vi "Exp_PopulateADCQualityControl.vi"(8 "error in (no error)":errorcluster, 10 "Control":refnum<vi>, 11 "LightField Automation in":refnum<class "LightField Automation.lvclass">) -> (0 "error out":errorcluster, 3 "LightField Automation out":refnum<class "LightField Automation.lvclass">)   [LabVIEW 2020, in "LightField Automation.lvclass"]
uses:
  LightField Automation.lvclass
  C:/Program Files/Princeton Instruments/LightField/PrincetonInstruments.LightFieldAddInSupportServices.dll
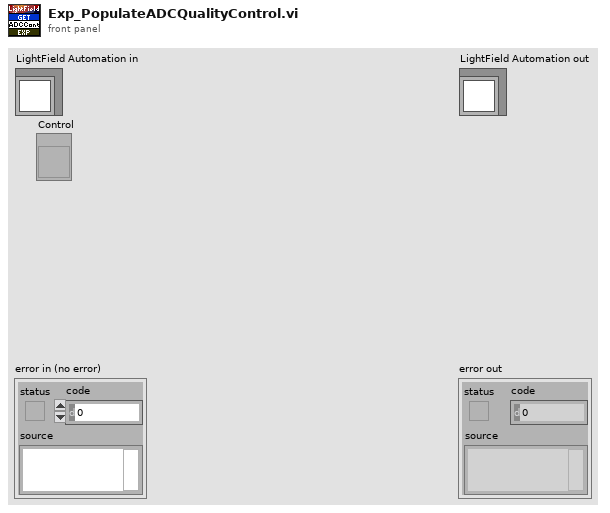
[diagram p1: front panel]
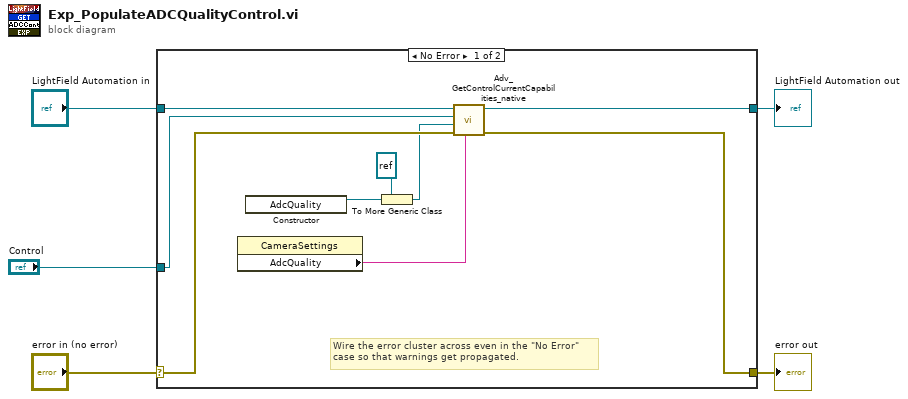
[diagram p0: block diagram]
diagram:
  n1 = case shown="No Error" "error in (no error)" {
    selector: "error in (no error)" -> [w12 w16]
    tunnel: [w11 w16] -> w4
    tunnel: [w14 w15] -> w2
    tunnel: "LightField Automation in" -> [w13 w15]
    tunnel: "Control" -> [w6 _]
    frame No Error {
      # "Wire the error cluster across even in the \"No Error\"\ncase so that warnings get propagated."
      n2 = property class="CameraSettings"() -> ("AdcQuality"=w8:string)  [unwired: 2 in, 2 out]
      n3 = constructor class="AdcQuality"() -> (reference out=w9:refnum<k24>)  [unwired: 3 in, 2 out]
      n4 = To More Generic Class(target class=refnum<k24> refnum, reference=w9) -> (generic class reference=w7:refnum<k24>)
      n5 = call "Adv_GetControlCurrentCapabilities_native.vi"("LightField Setting"=w8, "error in (no error)"=w12, "Enum Class"=w7, "Control"=w6, "LightField Automation in"=w13) -> ("error out"=w11:errorcluster, "LightField Automation out"=w14:refnum<class "LightField Automation.lvclass">)  [unwired: 5 in]
    }
    frame Error {
    }
  }
  "error out" <- w4
  "LightField Automation out" <- w2
